vi "PPMS Client.vi"(8 "error in (no error)":errorcluster, 9 "Data":variant, 10 "Command":string, 11 "instrument.PPMS2 in":refnum<class "instrument.PPMS.lvclass">) -> (0 "error out":errorcluster, 1 "Data out":variant, 2 "Command out":string, 3 "instrument.PPMS2 out":refnum<class "instrument.PPMS.lvclass">)   [LabVIEW 2016, in "instrument.PPMS.lvclass"]
uses:
  instrument.PPMS.lvclass
  C:/Program Files (x86)/National Instruments/LabVIEW 2016/user.lib/LevyLab/Levylab Instruments/SMOs/Instrument/Instrument.lvclass
  <userlib>/LevyLab/Levylab Instruments/SMOs/Instrument/Typedefs/SMO Configuration--Cluster.ctl
  <userlib>/LevyLab/Levylab Instruments/SMOs/Instrument/Typedefs/SMO RC Type--enum.ctl
  <userlib>/LevyLab/Levylab Instruments/SMOs/Instrument/Instrument.lvclass/Instrument.ctl
  <userlib>/LevyLab/Levylab Instruments/SMOs/Instrument/Instrument.lvclass
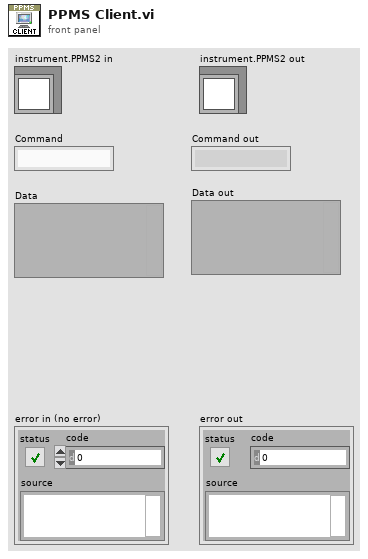
[diagram p1: front panel]
types:
  T1 = typedef "Instrument.lvclass/SMO RC Type--enum.ctl" = enum16{"RC", "STM", "ZMQ"}
  T2 = typedef "Instrument.lvclass/SMO Configuration--Cluster.ctl" = cluster{"Address":string, "Port":u16, "RC Type":T1}
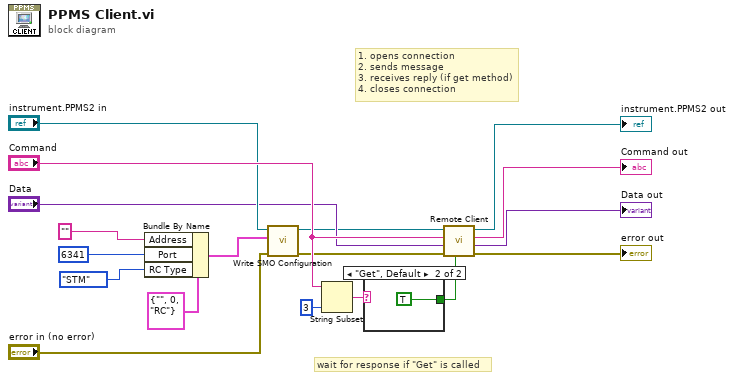
[diagram p0: block diagram]
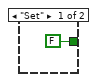
[diagram p2: hidden frame]
diagram:
  # "1. opens connection\n2. sends message\n3. receives reply (if get method)\n4. closes connection"
  # "wait for response if \"Get\" is called"
  n1 = Bundle By Name(cluster=T2 {"Address"="", "Port"=0, "RC Type"=enum."RC"} ("SMO"), "Address"="", "Port"=u16 6341, "RC Type"=SMO_RC_Type--enum."STM") -> (w1:T2)
  n2 = call <userlib>:"Write SMO Configuration.vi"("error in (no error)"="error in (no error)", "SMO"=w1, "Instrument in"="instrument.PPMS2 in") -> ("error out"=w6:errorcluster, "Instrument out"=w7:refnum<class "instrument.PPMS.lvclass">)  [unwired: 7 in]
  n3 = String Subset(string="Command", length (rest)=3 ("length (rest)")) -> (substring=w12:string)  [unwired: 1 in]
  n4 = case shown="\"Get\", Default" w12 {
    tunnel: [FALSE ("Wait for Response?") TRUE ("Wait for Response?")] -> w13
    frame "Set" {
    }
    frame "Get", Default {
    }
  }
  n5 = call <userlib>:"Remote Client.vi"("Wait for Response?"=w13, "error in (no error)"=w6, "Data"="Data", "Command"="Command", "Instrument in"=w7) -> ("error out"=→"error out":errorcluster, "Data out"=→"Data out":variant, "Command out"=→"Command out":string, "Instrument out"=→"instrument.PPMS2 out":refnum<class "instrument.PPMS.lvclass">)  [unwired: 3 in]
